vi "Get Data Marker Name [DM] Core.vi"(8 "error in (no error)":errorcluster, 9 "Name Buffer Size":i32 format="%.0g", 10 "Marker Index (1)":i32=1 format="%.0g", 11 "IVI_Fgen in":refnum<class "IVI_Fgen.lvclass">) -> (0 "error out":errorcluster, 2 "Marker Name":string, 3 "IVI_Fgen out":refnum<class "IVI_Fgen.lvclass">)   [LabVIEW 2015, in "IVI_Fgen.lvlib" / "IVI_Fgen.lvclass"]
doc: "This VI returns the repeated capability identifier for the data marker that corresponds to the one-based index you specify. If the value that you pass for the Index control is less than one or greater than the value of the data marker count, the VI returns an empty string in the Name control and returns an error.\n\nNote:\n\n(1) This VI is part of the IviFgenDataMarker [DM] extension group."
uses:
  IVI_Fgen.lvclass
  IVI_Fgen.lvclass/IVI_Fgen.ctl
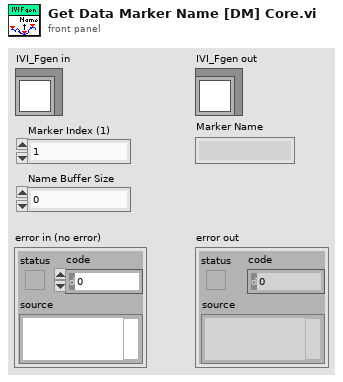
[diagram p1: front panel]
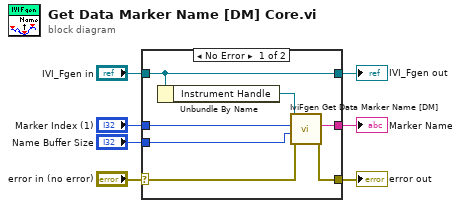
[diagram p0: block diagram]
diagram:
  n1 = case shown="No Error" "error in (no error)" {
    selector: "error in (no error)" -> [w12 w16]
    tunnel: [w11 w16] -> w6
    tunnel: [w14 w15] -> w4
    tunnel: "IVI_Fgen in" -> [w14 w15]
    tunnel: "Marker Index (1)" -> [w10 _]
    tunnel: "Name Buffer Size" -> [w9 _]
    tunnel: [w8 _] -> w1
    frame No Error {
      n2 = Unbundle By Name(w14) -> ("Instrument Handle"=w13:refnum<k15>)
      n3 = call <vilib>:"IviFgen Get Data Marker Name [DM].vi"("error in (no error)"=w12, "Name Buffer Size"=w9, "Marker Index (1)"=w10, "instrument handle"=w13) -> ("error out"=w11:errorcluster, "Marker Name"=w8:string)  [unwired: 5 in, 1 out]
    }
    frame Error {
    }
  }
  "error out" <- w6
  "IVI_Fgen out" <- w4
  "Marker Name" <- w1
